vi "ReadFromXML.vi"(8 "error in (no error)":errorcluster, 10 "XMLString in":string="<the_time>\n  <localTime>\n    <hours>0</hours>\n    <minutes>0</minutes>\n    <seconds>0</seconds>\n  </localTime>\n  <lst>\n    <hours>0</hours>\n    <minutes>0</minutes>\n    <seconds>0</seconds>\n  </lst>\n  <date>\n    <day>1</day>\n    <month>Jan</month>\n    <year>0</year>\n  </date>\n  <utc>\n    <hours>0</hours>\n    <minutes>0</minutes>\n    <seconds>0</seconds>\n  </utc>\n  <mjd>0</mjd>\n</the_time>") -> (0 "error out":errorcluster)   [LabVIEW 2022 SP3, in "TCSDataDefinitions.lvlib" / "TCSPublicStatus.lvlib" / "CurrentTimes.lvlib" / "CurrentTimes.lvclass"]
uses:
  CurrentTimes.lvclass
  CurrentTimes.lvclass/CurrentTimes.ctl
  ClockTimes/ClockTimes.lvclass
  <userlib>/Common/XML/XMLParser/XMLParser.lvclass
panel:
  out "time":timestamp
  out "CurrentTimes out":refnum<class "CurrentTimes.lvclass">
  in  "CurrentTimes in":refnum<class "CurrentTimes.lvclass">
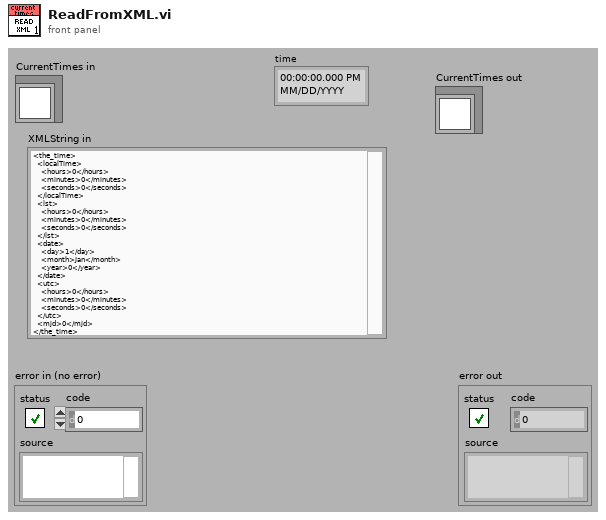
[diagram p1: front panel]
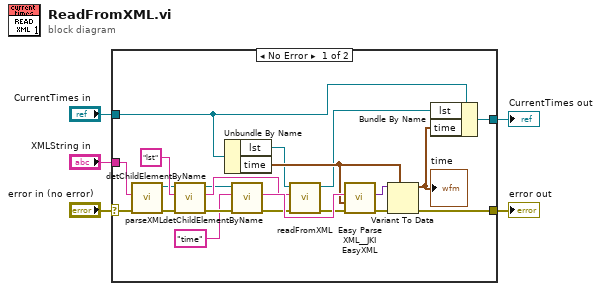
[diagram p0: block diagram]
diagram:
  n1 = case shown="No Error" "error in (no error)" {
    selector: "error in (no error)" -> [w25 w28]
    tunnel: [w8 w28] -> w4
    tunnel: [w20 w27] -> w1
    tunnel: "CurrentTimes in" -> [w21 w27]
    tunnel: "XMLString in" -> [w26 _]
    frame No Error {
      n2 = call <userlib>:"parseXML.vi"("error in (no error)"=w25, "XMLString in"=w26) -> ("error out"=w10:errorcluster, "Element out"=w7:refnum<class "XMLParser.lvclass">)  [unwired: 8 in]
      n3 = call <userlib>:"detChildElementByName.vi"("error in (no error)"=w10, "childName"="lst" ("ChildName"), "Element in"=w7) -> ("error out"=w24:errorcluster, "childXML"=w12:string, "Element out"=w6:refnum<class "XMLParser.lvclass">)  [unwired: 5 in, 1 out]
      n4 = Unbundle By Name(w21) -> ("lst"=w14:refnum<class "ClockTimes.lvclass">, "time"=w16:timestamp)
      n5 = call <userlib>:"detChildElementByName.vi"("error in (no error)"=w24, "childName"="time" ("ChildName"), "Element in"=w6) -> ("error out"=w9:errorcluster, "childXML"=w19:string)  [unwired: 5 in, 2 out]
      n6 = call-dynamic "readFromXML.vi"("error in (no error)"=w9, "XML in"=w12, "ClockTimes in"=w14) -> ("error out"=w13:errorcluster, "ClockTimes out"=w11:refnum<class "ClockTimes.lvclass">)  [unwired: 7 in]
      n7 = call <vilib>:"Easy Parse XML__JKI EasyXML.vi"("error in (no error)"=w13, "LabVIEW Data (Type)"=w16, "XML String"=w19) -> ("error out"=w17:errorcluster, "LabVIEW Data"=w18:variant)  [unwired: 7 in]
      n8 = Variant To Data(error in=w17, type=w16, Variant=w18) -> (data=w15:timestamp, error out=w8:errorcluster)
      "time" <- w15
      n9 = Bundle By Name(cluster=w21, "lst"=w11, "time"=w15) -> (w20:refnum<class "CurrentTimes.lvclass">)
    }
    frame Error {
    }
  }
  "error out" <- w4
  "CurrentTimes out" <- w1
